vi "Pressure Conversion.vi"(10 "Voltage":dbl, 11 "Baratron in":refnum<class "Baratron.lvclass">) -> (1 "Status Range":T1, 2 "Pressure":dbl)   [LabVIEW 2021, in "Baratron.lvclass"]
uses:
  Baratron.lvclass
  Status Range.ctl
  Baratron.lvclass/Baratron.ctl
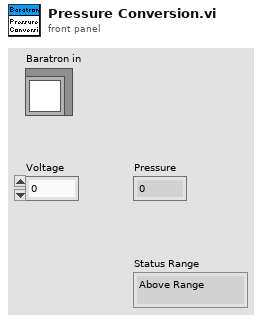
[diagram p1: front panel]
types:
  T1 = typedef "Baratron.lvclass/Status Range.ctl" = enum16{"Above Range", "Below Range", "Within Range"}
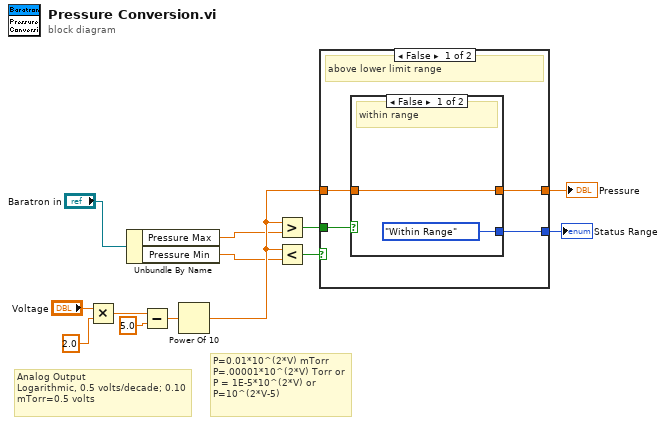
[diagram p0: block diagram]
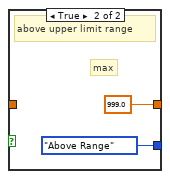
[diagram p2: hidden frame]
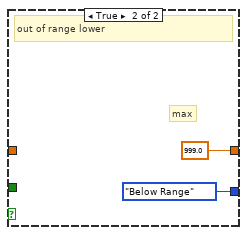
[diagram p3: hidden frame]
diagram:
  # "P=0.01*10^(2*V) mTorr\nP=.00001*10^(2*V) Torr or P = 1E-5*10^(2*V) or P=10^(2*V-5)"
  # "Analog Output\nLogarithmic, 0.5 volts/decade; 0.10 mTorr=0.5 volts"
  n1 = Multiply(x="Voltage", y=2.0) -> (x*y=w12:dbl)
  n2 = Unbundle By Name("Baratron in") -> ("Pressure Max"=w2:dbl, "Pressure Min"=w1:dbl)
  n3 = Subtract(x=w12, y=5.0) -> (x-y=w10:dbl)
  n4 = Power Of 10(x=w10) -> (10^x=w7:dbl)
  n5 = Greater?(x=w7, y=w2) -> (0:w6:bool)
  n6 = Less?(x=w7, y=w1) -> (x < y?=w5:bool)
  n7 = case shown="False" w5 {
    tunnel: w6 -> [w17 _]
    tunnel: w7 -> [w16 _]
    tunnel: [w15 999.0] -> w8
    tunnel: [w14 Status_Range."Below Range" ("Status Range")] -> w4
    frame False {
      # "above lower limit range"
      n8 = case shown="False" w17 {
        tunnel: w16 -> [w19 _]
        tunnel: [w19 999.0] -> w15
        tunnel: [Status_Range."Within Range" ("Status Range") Status_Range."Above Range" ("Status Range")] -> w14
        frame False {
          # "within range"
        }
        frame True {
          # "max"
          # "above upper limit range"
        }
      }
    }
    frame True {
      # "max"
      # "out of range lower"
    }
  }
  "Pressure" <- w8
  "Status Range" <- w4
